vi "Write I64 1D Value.vi"(8 "error in (no error)":errorcluster, 10 "I64 Value":i64[](array[numeric]), 11 "Numeric in":refnum<class "Abs_U64 Integer 1D.lvclass">) -> (0 "error out":errorcluster, 3 "Numeric out":refnum<class "Abs_U64 Integer 1D.lvclass">)   [LabVIEW 2021, in "Abs_U64 Integer 1D.lvclass"]
uses:
  Abs_U64 Integer 1D.lvclass
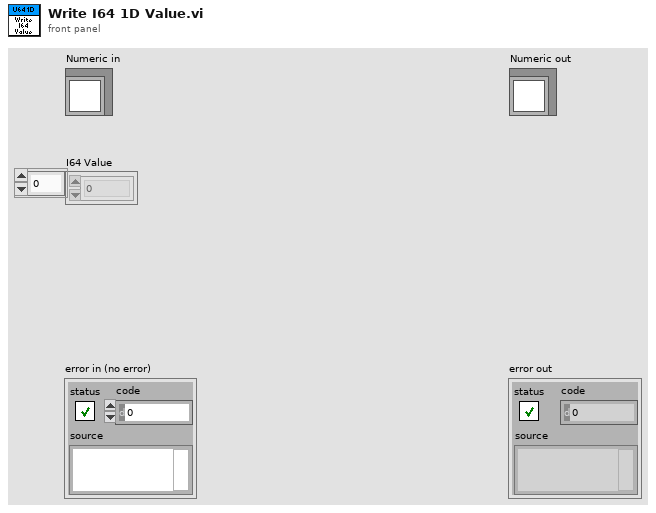
[diagram p1: front panel]
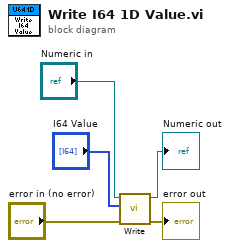
[diagram p0: block diagram]
diagram:
  n1 = call-dynamic "Write.vi"("error in (no error)"="error in (no error)", "Value"="I64 Value", "Double Float.lvclass in"="Numeric in") -> ("error out"=→"error out":errorcluster, "Double Float.lvclass out"=→"Numeric out":refnum<class "Abs_U64 Integer 1D.lvclass">)  [unwired: 7 in]
